vi "TTA_MATLAB_RFIC_Tile_Temp.vi"(11 "error in":errorcluster) -> (4 "Results":dbl[](array[numeric]), 6 "SuccessOp":bool[](array[boolean]), 8 "SuccessComm":bool[](array[boolean]), 15 "error out":errorcluster)   [LabVIEW 2016]
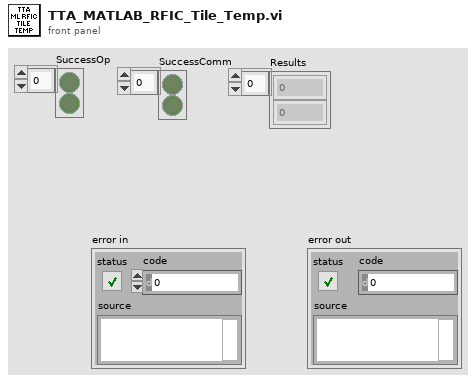
[diagram p1: front panel]
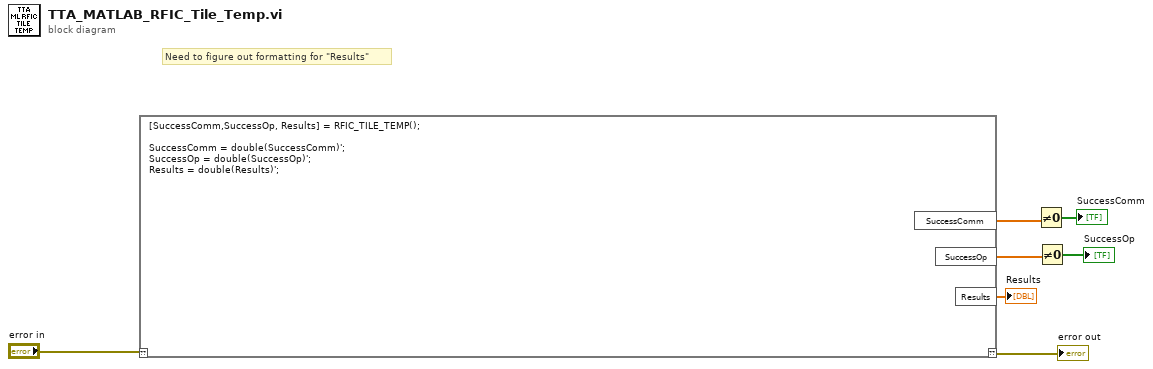
[diagram p0: block diagram]
diagram:
  # "Need to figure out formatting for \"Results\""
  n1 = script code="[SuccessComm,SuccessOp, Results] = RFIC_TILE_TEMP();\n\nSuccessComm = double(SuccessComm)';\nSuccessOp = double(SuccessOp)';\nResults = double(Results)';"("??"="error in") -> ("??"=→"error out":errorcluster, "SuccessComm"=w4:dbl[], "SuccessOp"=w3:dbl[], "Results"=→"Results":dbl[])
  n2 = Not Equal To 0?(x=w4) -> (x != 0?=→"SuccessComm":bool[])
  n3 = Not Equal To 0?(x=w3) -> (x != 0?=→"SuccessOp":bool[])
